vi "CRYGraph View Manager Socket Client.vi"(8 "pVI Ref":refnum<vi>, 9 "nData":i32, 10 "sData":string, 11 "sAction":string) -> ()   [LabVIEW 2013]
uses:
  Control/CRYPolar Property.ctl
  CRYCurveLibrary/Global/CRYCurve Library Global.vi
panel:
  in  "Polar Property":T1={"polar attributes"={"maximum"=2.0, "minimum"=0.0, "clip to min"=FALSE, "log"=FALSE, "grid color"=3381657, "plot color"=16711680, "fmt and prec"={"format"=enum."Decimal", "precision"=2}, "visible section"=4}, "Auto/Manual"=0, "Zero Adjust (deg)"=0, "Angle Increment (deg)"=0, "Mirror"=FALSE, "Auto Increment"=FALSE, "Total Rotatin (deg)"=0, "Discrete/Rannge"=0, "Show Name"=FALSE, "CurValues"=[], "CurIndex"=0, "CurColors"=[], "CurColors_Range"=[], "CurValues_Range"=[], "Pen"={"Width"=1, "Style"=enum."Solid"}, "BackgroundColor"=0} {"polar attributes"."minimum" format="%0.2f"; "polar attributes"."maximum" format="%0.2f"}
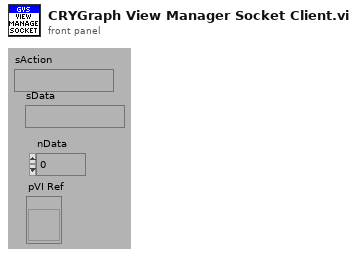
[diagram p1: front panel]
types:
  T1 = typedef "CRYPolar Property.ctl" = cluster{"polar attributes":cluster{"maximum":dbl, "minimum":dbl, "clip to min":bool, "log":bool, "grid color":u32, "plot color":u32, "fmt and prec":cluster{"format":enum8{"Decimal", "Scientific", "Engineering", "Binary", "Octal", "Hex"}, "precision":u8}, "visible section":u16}, "Auto/Manual":u16, "Zero Adjust (deg)":i32, "Angle Increment (deg)":i32, "Mirror":bool, "Auto Increment":bool, "Total Rotatin (deg)":i32, "Discrete/Rannge":u16, "Show Name":bool, "CurValues":dbl[], "CurIndex":u16, "CurColors":u32[], "CurColors_Range":u32[], "CurValues_Range":dbl[], "Pen":cluster{"Width":u16, "Style":enum32{"Solid", "Dash", "Dot", "DashDot", "DashDotDot"}}, "BackgroundColor":u32}
  T2 = typedef "CRYGraph Property.ctl" = cluster{"LegendShow":bool, "Legend Splitter Position":dbl, "Data Names":string[], "Item Symbols":i32[], "Color Array":u32[], "Flattened Plot Property":string, "CursorShow":bool, "Flattened Cursor Property":string, "Graph Number":i32, "Flattened Scale Property":string, "PreviewShow":bool, "MagnitudeShow":bool, "PaletteShow":bool, "XYShow":bool, "FrequencyShow":bool, "Frequency Splitter Position":dbl, "XYGraph Splitter Position":dbl, "Frequency Symbols":i32[], "LegendVScrollShow":bool, "FrequencyVScrollShow":bool, "PhaseShow":bool, "Title Name":string}
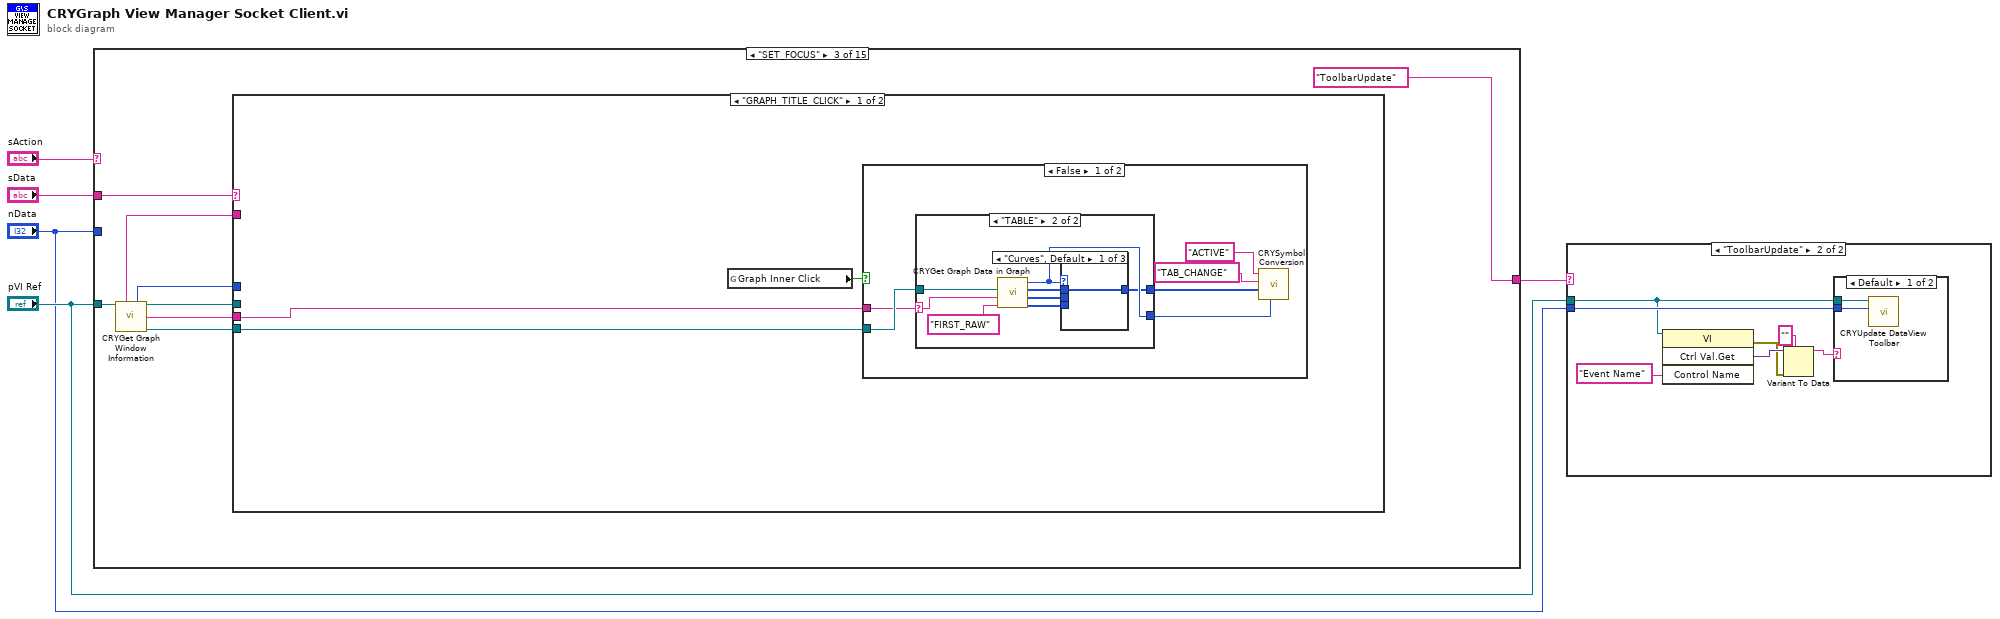
[diagram p0: block diagram]
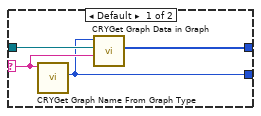
[diagram p6: hidden frame]
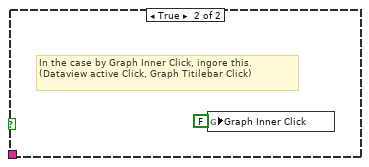
[diagram p9: hidden frame]
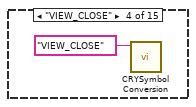
[diagram p11: hidden frame]
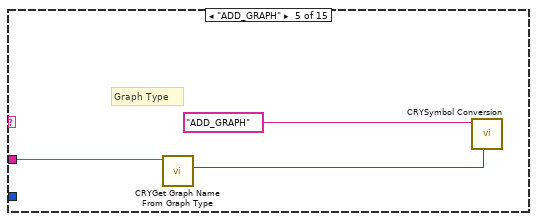
[diagram p12: hidden frame]
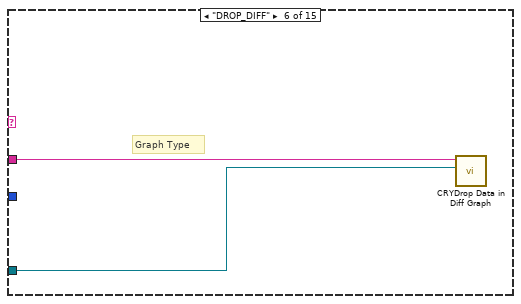
[diagram p13: hidden frame]
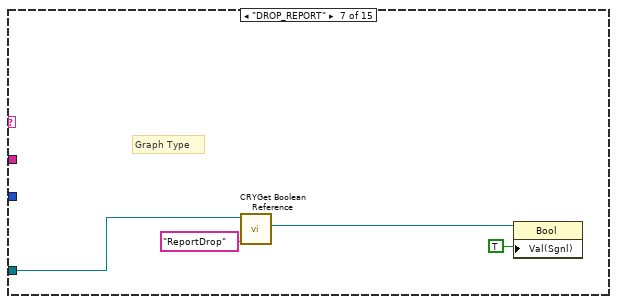
[diagram p14: hidden frame]
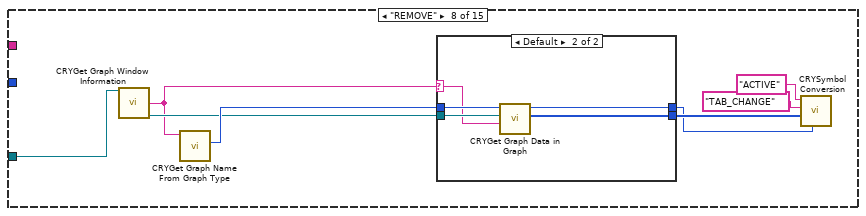
[diagram p15: hidden frame]
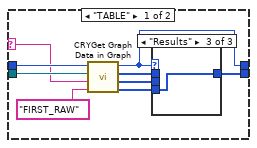
[diagram p16: hidden frame]
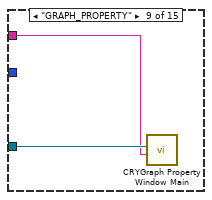
[diagram p19: hidden frame]
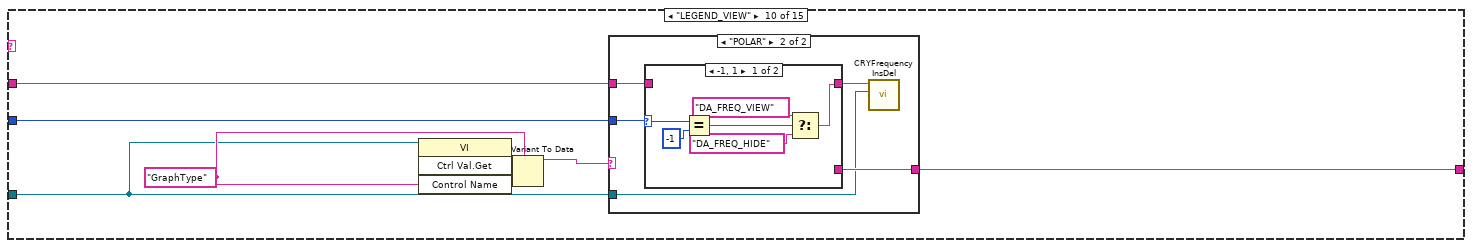
[diagram p20: hidden frame]
diagram:
  n1 = case shown="\"SET_FOCUS\"" "sAction" {
    selector: "sAction" -> [_ w6 _ _ _ _ _ _ _ _ _ _ w138 _ _]
    tunnel: "nData" -> [_ _ _ _ _ _ _ _ _ w82 w111 w125 w137 _ w160]
    tunnel: "sData" -> [_ _ w7 _ w43 w45 _ _ w75 w83 w113 w126 _ _ w161]
    tunnel: "pVI Ref" -> [_ _ w12 _ _ w44 w49 w57 w76 w77 w114 w127 w139 w148 w164]
    tunnel: [_ w6 "ToolbarUpdate" ("sData") _ _ _ _ _ _ w81 w110 w124 _ _ _] -> w3
    frame Default {
    }
    frame "ToolbarUpdate" {
    }
    frame "SET_FOCUS" {
      n2 = call "CRYGet Graph Window Information.vi"("pGraph VI In"=w12) -> ("Queue Name Out"=w9:string, "Graph Number Out"=w8:i32, "pGraph VI Out"=w10:refnum<vi>, "Graph Type Out"=w14:string, "Legend Ref Out"=w13:refnum<vi>)  [unwired: 4 in, 6 out]
      n3 = case shown="\"GRAPH_TITLE_CLICK\"" w7 {
        tunnel: w8 -> [_ _]
        tunnel: w9 -> [_ _]
        tunnel: w14 -> [w16 _]
        tunnel: w13 -> [w17 _]
        tunnel: w10 -> [_ _]
        frame "GRAPH_TITLE_CLICK" {
          n4 = global read "CRYCurve Library Global.vi" "Graph Inner Click"() -> (w15:bool)
          n5 = case shown="False" w15 {
            tunnel: w17 -> [w23 _]
            tunnel: w16 -> [w22 _]
            frame False {
              n6 = case shown="\"TABLE\"" w22 {
                selector: w22 -> [w26 w31]
                tunnel: w23 -> [w27 w30]
                tunnel: [w25 w29] -> w21
                tunnel: [w24 w28] -> w20
                frame Default {
                  n7 = call "CRYGet Graph Name From Graph Type.vi"("Graph Type"=w26) -> ("Type"=w25:enum16{"Curves", "Values", "Results", "WFM"})  [unwired: 9 in, 1 out]
                  n8 = call "CRYGet Graph Data in Graph.vi"("Graph Type"=w26, "Legend Refnum"=w27, "Type In"=w25) -> ("Rows"=w24:i32[])  [unwired: 1 in, 7 out]
                }
                frame "TABLE" {
                  n9 = call "CRYGet Graph Data in Graph.vi"("sOption"="FIRST_RAW", "Graph Type"=w31, "Legend Refnum"=w30) -> ("Result Rows"=w35:i32[], "Value Rows"=w34:i32[], "Rows"=w33:i32[], "Type Out"=w29:enum16{"Curves", "Values", "Results", "WFM"})  [unwired: 1 in, 4 out]
                  n10 = case shown="\"Curves\", Default" w29 {
                    tunnel: w33 -> [w36 _ _]
                    tunnel: w34 -> [_ w37 _]
                    tunnel: w35 -> [_ _ w38]
                    tunnel: [w36 w37 w38] -> w28
                    frame "Curves", Default {
                    }
                    frame "Values" {
                    }
                    frame "Results" {
                    }
                  }
                }
              }
              n11 = call "CRYSymbol Conversion.vi"("CurLib Tab Type"=w21, "nDatas"=w20, "sData"="TAB_CHANGE" ("sActin"), "sActin"="ACTIVE") -> ()  [unwired: 8 in]
            }
            frame True {
              # "In the case by Graph Inner Click, ingore this.\n(Dataview active Click, Graph Titilebar Click)"
              n12 = global write "CRYCurve Library Global.vi" "Graph Inner Click"(FALSE ("Graph Inner Click")) -> ()
            }
          }
        }
        frame Default {
          # "Graph inner Click"
        }
      }
    }
    frame "VIEW_CLOSE" {
      n13 = call "CRYSymbol Conversion.vi"("sActin"="VIEW_CLOSE") -> ()  [unwired: 11 in]
    }
    frame "ADD_GRAPH" {
      # "Graph Type"
      n14 = call "CRYGet Graph Name From Graph Type.vi"("Graph Type"=w43) -> ("Type"=w42:enum16{"Curves", "Values", "Results", "WFM"})  [unwired: 9 in, 1 out]
      n15 = call "CRYSymbol Conversion.vi"("CurLib Tab Type"=w42, "sActin"="ADD_GRAPH") -> ()  [unwired: 10 in]
    }
    frame "DROP_DIFF" {
      # "Graph Type"
      n16 = call "CRYDrop Data in Diff Graph.vi"("pGraph VI In"=w44, "Graph Type"=w45) -> ()  [unwired: 10 in]
    }
    frame "DROP_REPORT" {
      # "Graph Type"
      n17 = call "CRYGet Boolean Reference.vi"("Label Name"="ReportDrop", "VI Refnum"=w49) -> ("Boolean Ref"=w47:refnum<vi>)  [unwired: 7 in, 2 out]
      n18 = property class="Bool"(reference=w47, "Val(Sgnl)"=TRUE) -> ()  [unwired: 1 in, 2 out]
    }
    frame "REMOVE" {
      n19 = call "CRYGet Graph Window Information.vi"("pGraph VI In"=w57) -> ("Graph Type Out"=w50:string, "Legend Ref Out"=w54:refnum<vi>)  [unwired: 4 in, 9 out]
      n20 = call "CRYGet Graph Name From Graph Type.vi"("Graph Type"=w50) -> ("Type"=w55:enum16{"Curves", "Values", "Results", "WFM"})  [unwired: 9 in, 1 out]
      n21 = case shown="Default" w50 {
        selector: w50 -> [w64 w70]
        tunnel: w55 -> [w66 w74]
        tunnel: w54 -> [w65 w73]
        tunnel: [w58 w72] -> w53
        tunnel: [w59 w71] -> w51
        frame "TABLE" {
          n22 = call "CRYGet Graph Data in Graph.vi"("sOption"="FIRST_RAW", "Graph Type"=w64, "Legend Refnum"=w65, "Type In"=w66) -> ("Result Rows"=w60:i32[], "Value Rows"=w61:i32[], "Rows"=w62:i32[], "Type Out"=w59:enum16{"Curves", "Values", "Results", "WFM"})  [unwired: 4 out]
          n23 = case shown="\"Results\"" w59 {
            tunnel: w62 -> [w67 _ _]
            tunnel: w61 -> [_ w68 _]
            tunnel: w60 -> [_ _ w69]
            tunnel: [w67 w68 w69] -> w58
            frame "Curves", Default {
            }
            frame "Values" {
            }
            frame "Results" {
            }
          }
        }
        frame Default {
          n24 = call "CRYGet Graph Data in Graph.vi"("Graph Type"=w70, "Legend Refnum"=w73, "Type In"=w74) -> ("Rows"=w72:i32[], "Type Out"=w71:enum16{"Curves", "Values", "Results", "WFM"})  [unwired: 1 in, 6 out]
        }
      }
      n25 = call "CRYSymbol Conversion.vi"("CurLib Tab Type"=w51, "nDatas"=w53, "sData"="TAB_CHANGE" ("sActin"), "sActin"="ACTIVE") -> ()  [unwired: 8 in]
    }
    frame "GRAPH_PROPERTY" {
      n26 = call "CRYGraph Property Window Main.vi"("TabName"=w75, "pGraph VI In"=w76) -> ()  [unwired: 1 in, 9 out]
    }
    frame "LEGEND_VIEW" {
      w79 = "GraphType" ("Control Name")
      n27 = invoke class="VI" method="Ctrl Val.Get"(reference=w77, "Control Name"=w79) -> ("Get Control Value Variant"=w80:variant)  [unwired: 2 in, 3 out]
      n28 = Variant To Data(type=w79, Variant=w80) -> (data=w78:string)  [unwired: 1 in, 1 out]
      n29 = case shown="\"POLAR\"" w78 {
        tunnel: w83 -> [w88 w101]
        tunnel: w82 -> [w86 w99]
        tunnel: [w85 w98] -> w81
        tunnel: w77 -> [w84 w97]
        frame Default {
          n30 = case shown="-1, 1" w86 {
            selector: w86 -> [w89 _]
            tunnel: w88 -> [_ w96]
            tunnel: [w90 w96] -> w87
            tunnel: [_ "ToolbarUpdate" ("sData")] -> w85
            frame -1, 1 {
              n31 = Equal?(x=w89, y=-1) -> (x = y?=w93:bool)
              n32 = Select(t="DA_LEG_VIEW", s=w93, f="DA_LEG_HIDE" ("sData")) -> (s? t:f=w90:string)
            }
            frame Default {
            }
          }
          n33 = call "CRYData View Legend InsDel.vi"("Graph VI Ref"=w84, "sAction"=w87) -> ()  [unwired: 3 in, 7 out]
        }
        frame "POLAR" {
          n34 = case shown="-1, 1" w99 {
            selector: w99 -> [w102 _]
            tunnel: w101 -> [_ w109]
            tunnel: [w103 w109] -> w100
            tunnel: [_ "ToolbarUpdate" ("sData")] -> w98
            frame -1, 1 {
              n35 = Equal?(x=w102, y=-1) -> (x = y?=w106:bool)
              n36 = Select(t="DA_FREQ_VIEW", s=w106, f="DA_FREQ_HIDE" ("sData")) -> (s? t:f=w103:string)
            }
            frame Default {
            }
          }
          n37 = call "CRYFrequency InsDel.vi"("Graph VI Ref"=w97, "sAction"=w100) -> ()  [unwired: 10 in]
        }
      }
    }
    frame "CURSOR_VIEW" {
      n38 = case shown="-1, 1" w111 {
        selector: w111 -> [w115 _]
        tunnel: w113 -> [_ w122]
        tunnel: [w116 w122] -> w112
        tunnel: [_ "ToolbarUpdate" ("sData")] -> w110
        frame -1, 1 {
          n39 = Equal?(x=w115, y=-1) -> (x = y?=w119:bool)
          n40 = Select(t="DA_CUR_VIEW", s=w119, f="DA_CUR_HIDE" ("sData")) -> (s? t:f=w116:string)
        }
        frame Default {
        }
      }
      n41 = call "CRYCursor InsDel.vi"("Graph VI Ref"=w114, "sAction"=w112) -> ()  [unwired: 10 in]
    }
    frame "PREVIEW_VIEW" {
      n42 = case shown="Default" w125 {
        selector: w125 -> [w128 _]
        tunnel: w126 -> [_ w135]
        tunnel: [w129 w135] -> w123
        tunnel: [_ "ToolbarUpdate" ("sData")] -> w124
        frame -1, 1 {
          n43 = Equal?(x=w128, y=-1) -> (x = y?=w132:bool)
          n44 = Select(t="DA_PRE_VIEW", s=w132, f="DA_PRE_HIDE" ("sData")) -> (s? t:f=w129:string)
        }
        frame Default {
        }
      }
      n45 = call "CRYPreview InsDel.vi"("Graph VI Ref"=w127, "sAction"=w123) -> ()  [unwired: 10 in]
    }
    frame "X_AUTOSCALE", "Y1_AUTOSCALE", "Y2_AUTOSCALE" {
      n46 = case shown="-1, 1" w137 {
        selector: w137 -> [w140 _]
        tunnel: [w141 "NONE" ("sData")] -> w136
        frame -1, 1 {
          n47 = Equal?(x=w140, y=1) -> (x = y?=w144:bool)
          n48 = Select(t="DA_SCA_ON", s=w144, f="DA_SCA_OFF" ("sData")) -> (s? t:f=w141:string)
        }
        frame Default {
        }
      }
      n49 = call "CRYAutoScale Change.vi"("sOption"=w136, "Graph VI Ref"=w139, "sAction"=w138) -> ()  [unwired: 9 in]
    }
    frame "CURSOR_PROPERTY" {
      n50 = flat-sequence {
        tunnel: w148 -> [w153]
        tunnel: [w149] -> w147
        tunnel: w147 -> [w154]
        frame #0 {
          n51 = call "CRYGet String Reference.vi"("Label Name"="PropertyTab", "VI Refnum"=w153) -> ("String Ref Out"=w151:refnum<vi>, "VI Refnum Out"=w149:refnum<vi>)  [unwired: 7 in, 1 out]
          n52 = property class="Str"(reference=w151, "Value"="Cursor" ("Tab Name")) -> ()  [unwired: 1 in, 2 out]
        }
        frame #1 {
          n53 = call "CRYGet Boolean Reference.vi"("Label Name"="OpenProperty", "VI Refnum"=w154) -> ("Boolean Ref"=w156:refnum<vi>)  [unwired: 7 in, 2 out]
          n54 = property class="Bool"(reference=w156, "Val(Sgnl)"=TRUE) -> ()  [unwired: 1 in, 2 out]
        }
      }
    }
    frame "ADD_DOC" {
      n55 = call "CRYGraph View Socket Client.vi"("sOption"="FROM_GRAPHNUMBER", "nData"=w160, "sData"=w161, "sAction"="GET_GRAPHWINDOW") -> ("bResult Out"=w158:bool, "pVI Out"=w159:refnum<vi>)  [unwired: 4 in, 2 out]
      n56 = case shown="True" w158 {
        tunnel: w164 -> [_ w172]
        tunnel: w159 -> [_ w171]
        frame False {
        }
        frame True {
          n57 = invoke class="VI" method="Ctrl Val.Get"(reference=w171, "Control Name"="GraphType") -> ("Get Control Value Variant"=w168:variant)  [unwired: 2 in, 3 out]
          n58 = Variant To Data(type="", Variant=w168) -> (data=w166:string)  [unwired: 1 in, 1 out]
          n59 = call "CRYGraph Get.vi"("pGraph VI In"=w171) -> ("Graph Cluster"=w170:T2)  [unwired: 10 in]
          n60 = case shown="\"POLAR\"" w166 {
            tunnel: w170 -> [w173 w176]
            tunnel: [w173 w174] -> w169
            frame Default {
            }
            frame "POLAR" {
              n61 = Unbundle By Name(w176) -> ("Flattened Plot Property"=w185:string)
              n62 = call "CRYUnflatten Graph Property.vi"("Cluster Name"="POLAR", "Flatten Graph Property"=w185) -> ("Flatten Graph Property Out"=w182:string)  [unwired: 7 in, 2 out]
              n63 = Unflatten From String(type="Polar Property", binary string=w182) -> (value=w181:T1)  [unwired: 1 in, 4 out]
              n64 = Bundle By Name(cluster=w181, "BackgroundColor"=u32 16777226) -> (w179:T1)
              n65 = Flatten To String(anything=w179) -> (data string=w178:string)  [unwired: 3 in, 2 out]
              n66 = call "CRYFlatten Graph Property.vi"("Cluster Name"="POLAR", "GraphProperty"=w178) -> ("GraphProperty Flattened"=w175:string)  [unwired: 9 in]
              n67 = Bundle By Name(cluster=w176, "Flattened Plot Property"=w175) -> (w174:T2)
            }
          }
          n68 = call "CRYGraph Set.vi"("Graph Property"=w169, "pGraph VI In"=w172) -> ()  [unwired: 10 in]
        }
      }
    }
  }
  n69 = case shown="\"ToolbarUpdate\"" w3 {
    tunnel: "pVI Ref" -> [_ w188]
    tunnel: "nData" -> [_ w192]
    frame Default {
    }
    frame "ToolbarUpdate" {
      n70 = invoke class="VI" method="Ctrl Val.Get"(reference=w188, "Control Name"="Event Name") -> (error out=w190:errorcluster, "Get Control Value Variant"=w191:variant)  [unwired: 2 in, 2 out]
      n71 = Variant To Data(error in=w190, type="" ("Control Name"), Variant=w191) -> (data=w186:string)  [unwired: 1 out]
      n72 = case shown="Default" w186 {
        tunnel: w192 -> [w194 _]
        tunnel: w188 -> [w193 _]
        frame Default {
          n73 = call "CRYUpdate DataView Toolbar.vi"("nData"=w194, "pVI"=w193) -> ()  [unwired: 10 in]
        }
        frame "ViewReport" {
        }
      }
    }
  }
